vi "Create ParentClass.vi"(5 "ParentClass in":refnum<class "ParentClass.lvclass">, 8 "error in (no error)":errorcluster, 11 "Numeric":dbl) -> (0 "error out":errorcluster, 3 "ParentClass":refnum<class "ParentClass.lvclass">)   [LabVIEW 2017, in "TestLibrary.lvlib" / "ParentClass.lvclass"]
uses:
  ParentClass.lvclass
  ParentClass.lvclass/ParentClass.ctl
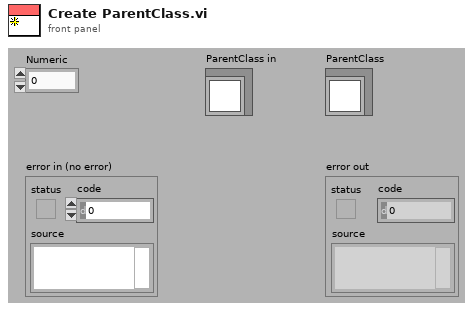
[diagram p1: front panel]
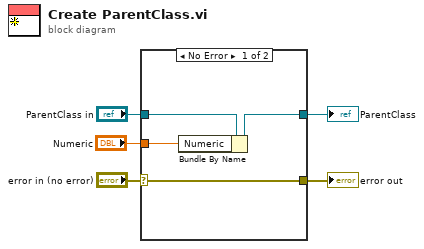
[diagram p0: block diagram]
diagram:
  n1 = case shown="No Error" "error in (no error)" {
    selector: "error in (no error)" -> [w9 w11]
    tunnel: [w9 w11] -> w4
    tunnel: [w7 w10] -> w2
    tunnel: "ParentClass in" -> [w8 w10]
    tunnel: "Numeric" -> [w6 _]
    frame No Error {
      n2 = Bundle By Name(cluster=w8, "Numeric"=w6) -> (w7:refnum<class "ParentClass.lvclass">)
    }
    frame Error {
    }
  }
  "error out" <- w4
  "ParentClass" <- w2
